vi "Test Depth and Color.vi"() -> ()   [LabVIEW 2017]
uses:
  <vilib>/addons/RealSense/libRealSense3.lvlib
  <vilib>/vision/NI_Vision_Development_Module.lvlib
  <vilib>/addons/RealSense/realsense-d.dll
panel:
  out "motion result":i32
  out "ms":u32
  out "intrin out":T1 {"model" items=["RS_DISTORTION_NONE", "RS_DISTORTION_MODIFIED_BROWN_CONRADY", "RS_DISTORTION_INVERSE_BROWN_CONRADY", "RS_DISTORTION_FTHETA", "RS_DISTORTION_BROWN_CONRADY", "RS_DISTORTION_COUNT"]}
  out "Image 2":T2(plugin-control)
  out "Image":T2(plugin-control)
  out "error out":errorcluster
  in  "stop":bool
  out "device count":i32
  # "All errors are #1, string is good"
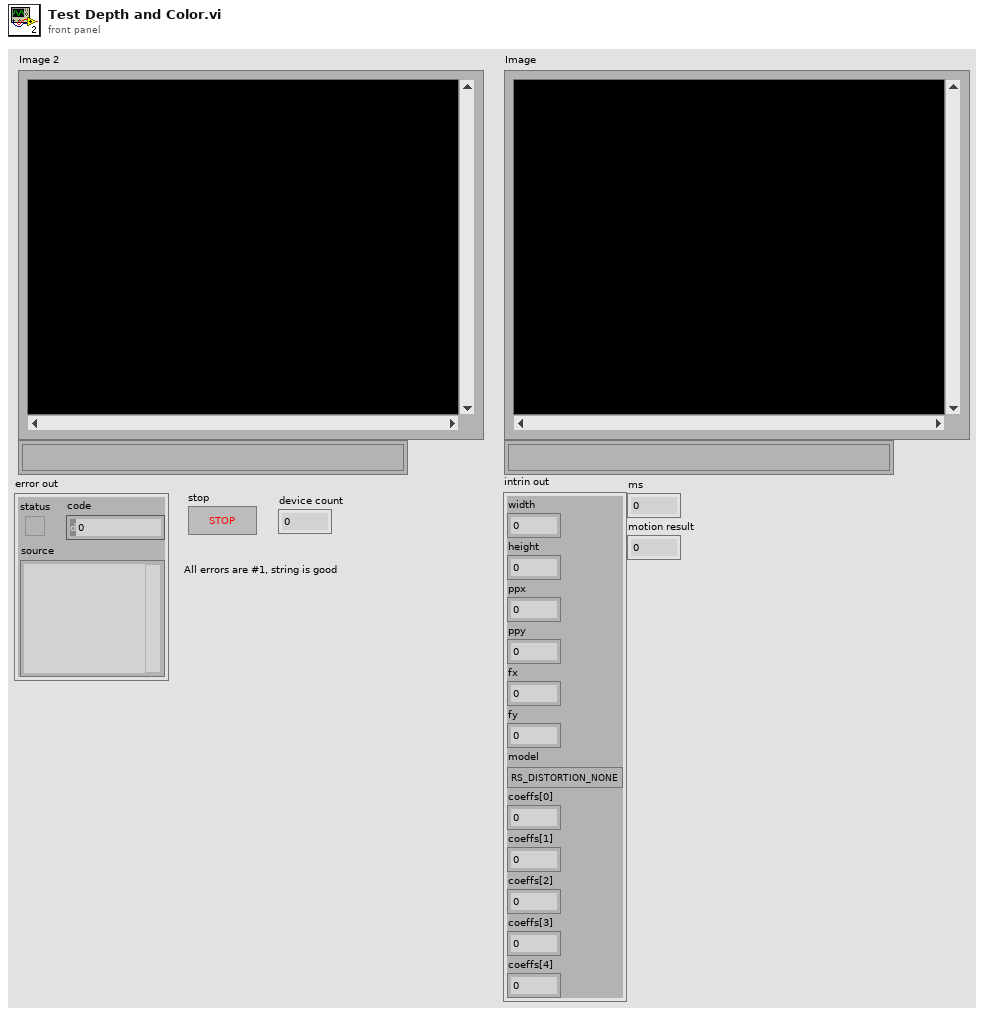
[diagram p1: front panel]
types:
  T1 = cluster{"width":i32, "height":i32, "ppx":sgl, "ppy":sgl, "fx":sgl, "fy":sgl, "model":u32, "coeffs[0]":sgl, "coeffs[1]":sgl, "coeffs[2]":sgl, "coeffs[3]":sgl, "coeffs[4]":sgl}
  T2 = typedef "IMAQ Image.ctl" = refnum<image>
  T3 = typedef "Image Type" = u32
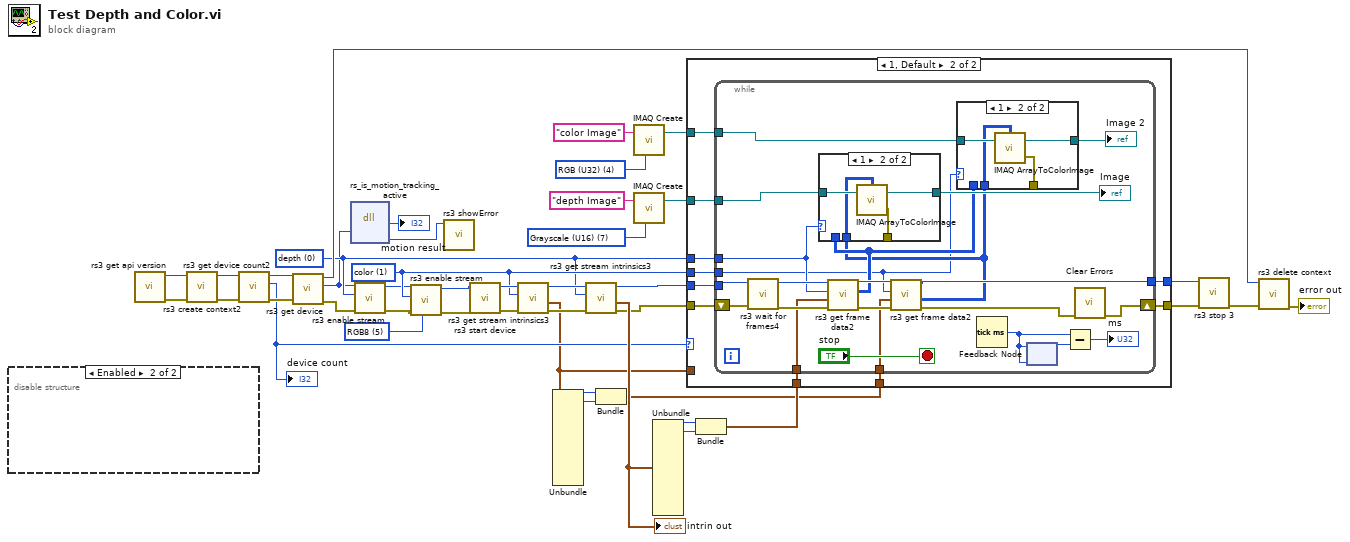
[diagram p0: block diagram]
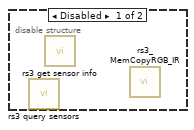
[diagram p2: hidden frame]
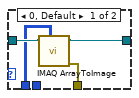
[diagram p4: hidden frame]
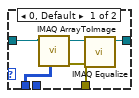
[diagram p5: hidden frame]
diagram:
  w13 = T3 4 items=["Grayscale (U8)", "Grayscale (I16)", "Grayscale (SGL)", "Complex (CSG)", "RGB (U32)", "HSL (U32)", "RGB (U64)", "Grayscale (U16)"] ("Image Type")
  w18 = u16 5 items=["any", "Depth16", "Disparity16", "f32XYZ", "YUV", "RGB8", "BGR8", "RGBA8", "BGRA8", "Y8", "Y16", "Raw10", "Raw16", "Raw8"] ("format")
  w10 = u16 1 items=["depth", "color", "inf 1", "inf 2"] ("stream type")
  w9 = u16 0 items=["depth", "color", "inf 1", "inf 2"] ("stream type")
  w23 = T3 7 items=["Grayscale (U8)", "Grayscale (I16)", "Grayscale (SGL)", "Complex (CSG)", "RGB (U32)", "HSL (U32)", "RGB (U64)", "Grayscale (U16)"] ("Image Type")
  n1 = disable-structure shown="Enabled" {
    frame Disabled {
      n2 = call <vilib>:"rs3 query sensors.vi"() -> ()  [unwired: 9 in, 3 out]
      n3 = call <vilib>:"rs3 get sensor info.vi"() -> ()  [unwired: 8 in, 4 out]
      n4 = call <vilib>:"rs3_MemCopyRGB_IR.vi"() -> ()  [unwired: 14 in, 2 out]
    }
    frame Enabled {
    }
  }
  n5 = call <vilib>:"rs3 get api version.vi"() -> ("error out"=w35:errorcluster, "version"=w43:i32)  [unwired: 10 in]
  n6 = call <vilib>:"rs3 create context2.vi"("error in (no error)"=w35, "version"=w43) -> ("error out"=w34:errorcluster, "context"=w42:u32)  [unwired: 8 in]
  n7 = call <vilib>:"rs3 get device count2.vi"("error in"=w34, "context"=w42) -> ("error out"=w33:errorcluster, "count"=w26:i32, "context"=w41:u32)  [unwired: 7 in]
  "device count" <- w26
  n8 = call <vilib>:"rs3 get device.vi"("error in"=w33, "context"=w41) -> ("error out"=w32:errorcluster, "device"=w2:u32, "context"=w36:u64)  [unwired: 7 in]
  n9 = dll-call lib="C:/Program Files (x86)/National Instruments/LabVIEW 2017/vi.lib/addons/RealSense/realsense-d.dll" fn="rs_is_motion_tracking_active"("device"=w2) -> ("flags"=→"motion result":i32, "error"=w1:u64)  [unwired: 5 in, 2 out]
  n10 = call <vilib>:"rs3 enable stream.vi"("error in"=w32, "stream type"=w9, "device"=w2) -> ("error out"=w19:errorcluster, "device"=w4:u32)  [unwired: 7 in]
  n11 = call <vilib>:"rs3 enable stream.vi"("format"=w18, "error in"=w19, "stream type"=w10, "device"=w4) -> ("error out"=w20:errorcluster, "device"=w21:u32)  [unwired: 6 in]
  n12 = call <vilib>:"rs3 showError.vi"("error"=w1) -> ()  [unwired: 6 in, 5 out]
  n13 = call <vilib>:"rs3 start device.vi"("error in"=w20, "device"=w21) -> ("error out"=w16:errorcluster, "device"=w17:u64)  [unwired: 8 in]
  n14 = call <vilib>:"rs3 get stream intrinsics3.vi"("error in (no error)"=w16, "stream type"=w10, "device in"=w17) -> ("error out"=w15:errorcluster, "intrin out"=w7:T1, "device out"=w14:u64)  [unwired: 6 in]
  n15 = Unbundle(w7) -> ("width"=w6:i32, "height"=w8:i32)  [unwired: 10 out]
  n16 = call <vilib>:"rs3 get stream intrinsics3.vi"("error in (no error)"=w15, "stream type"=w9, "device in"=w14) -> ("error out"=w31:errorcluster, "intrin out"=w39:T1, "device out"=w40:u64)  [unwired: 6 in]
  "intrin out" <- w39
  n17 = Bundle("width"=w6, "height"=w8) -> (w5:cluster{"width":i32, "height":i32})  [unwired: 1 in]
  n18 = call "IMAQ Create"("Image Name"="color Image", "Image Type"=w13) -> ("New Image"=w11:T2)  [unwired: 3 in, 1 out]
  n19 = call "IMAQ Create"("Image Name"="depth Image", "Image Type"=w23) -> ("New Image"=w22:T2)  [unwired: 3 in, 1 out]
  n20 = Unbundle(w39) -> ("width"=w29:i32, "height"=w28:i32)  [unwired: 10 out]
  n21 = Bundle("width"=w29, "height"=w28) -> (w27:cluster{"width":i32, "height":i32})  [unwired: 1 in]
  n22 = case shown="1, Default" w26 {
    tunnel: w40 -> [w45 w55]
    tunnel: [w45 w54] -> w38
    tunnel: w31 -> [w44 w53]
    tunnel: [w44 w52] -> w30
    tunnel: w27 -> [_ w51]
    tunnel: w22 -> [_ w50]
    tunnel: w9 -> [_ w49]
    tunnel: w7 -> [_ _]
    tunnel: w11 -> [_ w48]
    tunnel: w10 -> [_ w47]
    tunnel: w5 -> [_ w46]
    frame 0 {
    }
    frame 1, Default {
      n23 = while {
        tunnel: w55 -> [w76]
        tunnel: [w69] -> w54
        shift-right: [w72] -> w52
        shift-left: w53 -> [w74]
        tunnel: w51 -> [w73]
        tunnel: w50 -> [w64]
        tunnel: w49 -> [w61]
        tunnel: w48 -> [w71]
        tunnel: w47 -> [w60]
        tunnel: w46 -> [w59]
        stop <- "stop" stop-if-true
        n24 = call <vilib>:"rs3 wait for frames4.vi"("error in (no error)"=w74, "device in"=w76) -> ("error out"=w78:errorcluster, "device out"=w75:u64)  [unwired: 8 in]
        n25 = call <vilib>:"rs3 get frame data2.vi"("error in (no error)"=w78, "size"=w73, "stream type"=w61, "device in"=w75) -> ("error out"=w68:errorcluster, "2D Depth Output"=w63:u16[][], "device out"=w70:u64)  [unwired: 4 in, 1 out]
        n26 = call <vilib>:"rs3 get frame data2.vi"("error in (no error)"=w68, "size"=w59, "stream type"=w60, "device in"=w70) -> ("error out"=w67:errorcluster, "2D Color Output"=w62:u32[][], "device out"=w69:u64)  [unwired: 4 in, 1 out]
        n27 = case shown="1" w61 {
          tunnel: w64 -> [w81 w86]
          tunnel: [w79 w85] -> w65
          tunnel: [w82 w84] -> _
          tunnel: w63 -> [w80 _]
          tunnel: w62 -> [_ w83]
          frame 0, Default {
            n28 = call "IMAQ ArrayToImage"("Image Pixels (U16)"=w80, "Image"=w81) -> ("error out"=w82:errorcluster, "Image Out"=w79:T2)  [unwired: 8 in]
          }
          frame 1 {
            n29 = call "IMAQ ArrayToColorImage"("Image Pixels (U32)"=w83, "Image"=w86) -> ("Image Out"=w85:T2, "error out"=w84:errorcluster)  [unwired: 3 in]
          }
        }
        "Image" <- w65
        n30 = case shown="1" w60 {
          tunnel: w71 -> [w88 w95]
          tunnel: [w91 w94] -> w66
          tunnel: [w89 w93] -> _
          tunnel: w63 -> [w87 _]
          tunnel: w62 -> [_ w92]
          frame 0, Default {
            n31 = call "IMAQ ArrayToImage"("Image Pixels (Float)"=w87, "Image"=w88) -> ("error out"=w89:errorcluster, "Image Out"=w90:T2)  [unwired: 8 in]
            n32 = call "IMAQ Equalize"("Image Src"=w90) -> ("Image Dst Out"=w91:T2)  [unwired: 9 in, 1 out]
          }
          frame 1 {
            n33 = call "IMAQ ArrayToColorImage"("Image Pixels (U32)"=w92, "Image"=w95) -> ("Image Out"=w94:T2, "error out"=w93:errorcluster)  [unwired: 3 in]
          }
        }
        "Image 2" <- w66
        n34 = Tick Count (ms)() -> (millisecond timer value=w57:u32)
        n35 = feedback-in #1(w57) -> ()
        n36 = feedback #1(w57) -> (w58:u32)
        n37 = Subtract(x=w57, y=w58) -> (x-y=→"ms":u32)
        n38 = call <vilib>:"Clear Errors.vi"("error in (no error)"=w67) -> ("error out"=w72:errorcluster)  [unwired: 5 in, 1 out]
      }
    }
  }
  n39 = call <vilib>:"rs3 stop 3.vi"("error in (no error)"=w30, "device"=w38) -> ("error out"=w37:errorcluster)  [unwired: 8 in, 1 out]
  n40 = call <vilib>:"rs3 delete context.vi"("error in (no error)"=w37, "context"=w36) -> ("error out"=→"error out":errorcluster)  [unwired: 9 in]
